vi "Unreserve Sessions Wrapper.vi"(8 "error in":errorcluster, 11 "request data":T2) -> (0 "error out":errorcluster, 3 "response data":T1)   [LabVIEW 2020, in "Plug-In SDK Session Management V1.lvlib" / "Session Reservation.lvclass"]
uses:
  Session Reservation.lvclass
  gRPC/Generated APIs/ni/measurementlink/sessionmanagement/v1/RPC Messages/ni_measurementlink_sessionmanagement_v1_UnreserveSessionsRequest.ctl
  gRPC/Generated APIs/ni/measurementlink/sessionmanagement/v1/RPC Messages/ni_measurementlink_sessionmanagement_v1_SessionInformation.ctl
  gRPC/Generated APIs/ni/measurementlink/sessionmanagement/v1/RPC Messages/nidevice_grpc_Session.ctl
  gRPC/Generated APIs/ni/measurementlink/sessionmanagement/v1/RPC Messages/ni_measurementlink_sessionmanagement_v1_ChannelMapping.ctl
  gRPC/Generated APIs/ni/measurementlink/sessionmanagement/v1/RPC Messages/ni_measurementlink_sessionmanagement_v1_UnreserveSessionsResponse.ctl
  Discovery V1/TypeDefs/gRPC Client Cache FGV Action.ctl
  Discovery V1/Plug-In SDK Discovery V1.lvlib
  gRPC/Generated APIs/ni/measurementlink/sessionmanagement/v1/ni.measurementlink.sessionmanagement.v1.lvlib
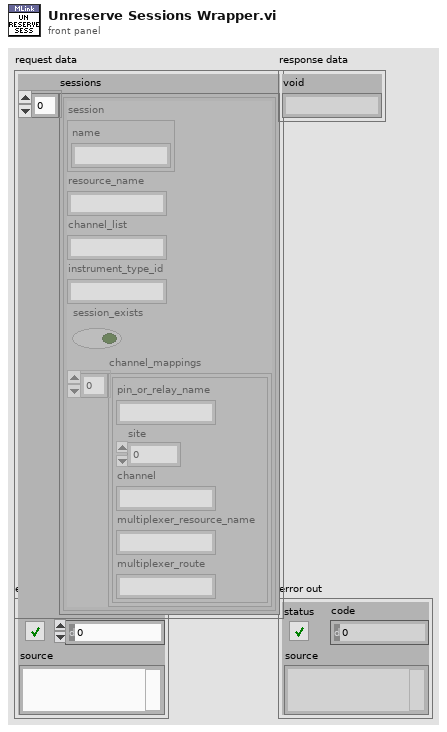
[diagram p1: front panel]
types:
  T1 = typedef "ni.measurementlink.sessionmanagement.v1.lvlib/ni_measurementlink_sessionmanagement_v1_UnreserveSessionsResponse.ctl" = cluster{"void":string}
  T2 = typedef "ni.measurementlink.sessionmanagement.v1.lvlib/ni_measurementlink_sessionmanagement_v1_UnreserveSessionsRequest.ctl" = cluster{"sessions":T3[]}
  T3 = typedef "ni.measurementlink.sessionmanagement.v1.lvlib/ni_measurementlink_sessionmanagement_v1_SessionInformation.ctl" = cluster{"session":T4, "resource_name":string, "channel_list":string, "instrument_type_id":string, "session_exists":bool, "channel_mappings":T5[]}
  T4 = typedef "ni.measurementlink.sessionmanagement.v1.lvlib/nidevice_grpc_Session.ctl" = cluster{"name":string}
  T5 = typedef "ni.measurementlink.sessionmanagement.v1.lvlib/ni_measurementlink_sessionmanagement_v1_ChannelMapping.ctl" = cluster{"pin_or_relay_name":string, "site":i32, "channel":string, "multiplexer_resource_name":string, "multiplexer_route":string}
  T6 = typedef "Plug-In SDK Discovery V1.lvlib/gRPC Client Cache FGV Action.ctl" = enum16{"Get Client", "Recreate Client", "Destroy Client", "Update ClusterId"}
  T7 = typedef "grpc-lvsupport-release.lvlib/grpcId.ctl" = u64
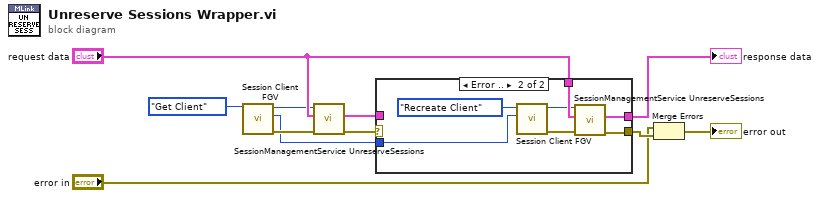
[diagram p0: block diagram]
diagram:
  n1 = call "Session Client FGV.vi"("action"=gRPC_Client_Cache_FGV_Action."Get Client") -> ("error out"=w9:errorcluster, "unique id out"=w4:u64, "grpc client id"=w5:T7)  [unwired: 8 in]
  n2 = call "SessionManagementService UnreserveSessions.vi"("error in"=w9, "Request Data"="request data", "gRPC ID"=w5) -> ("error out"=w8:errorcluster, "Response Data"=w6:T1)  [unwired: 6 in, 1 out]
  n3 = case shown="Error .." w8 {
    selector: w8 -> [w13 _]
    tunnel: [w13 w18] -> w2
    tunnel: [w12 w17] -> w10
    tunnel: w6 -> [w12 _]
    tunnel: "request data" -> [_ w16]
    tunnel: w4 -> [_ w15]
    frame No Error {
    }
    frame Error {
      n4 = call "Session Client FGV.vi"("unique id in"=w15, "action"=gRPC_Client_Cache_FGV_Action."Recreate Client") -> ("error out"=w19:errorcluster, "grpc client id"=w14:T7)  [unwired: 7 in, 1 out]
      n5 = call "SessionManagementService UnreserveSessions.vi"("error in"=w19, "Request Data"=w16, "gRPC ID"=w14) -> ("error out"=w18:errorcluster, "Response Data"=w17:T1)  [unwired: 6 in, 1 out]
    }
  }
  "response data" <- w10
  n6 = Merge Errors("error in", w2) -> (→"error out":errorcluster)
